vi "Write Motors with Encoders Config.vi"(8 "error in (no error)":errorcluster, 10 "Motors with Encoders Config":T1={"Counts  Per Revolution"=0, "Invert Encoder Direction"=FALSE, "Diameter of Revolution"=0.0, "Max RPM"=0.0, "Encoder Control"=TRUE}, 11 "Motors with Encoders in":refnum<class "Motors with Encoders.lvclass">) -> (0 "error out":errorcluster, 3 "Motors with Encoders out":refnum<class "Motors with Encoders.lvclass">)   [LabVIEW 2014, in "Motors with Encoders.lvlib" / "Motors with Encoders.lvclass"]
uses:
  Motors with Encoders.lvclass
  Motors with Encoders Config.ctl
  Motors with Encoders.lvclass/Motors with Encoders.ctl
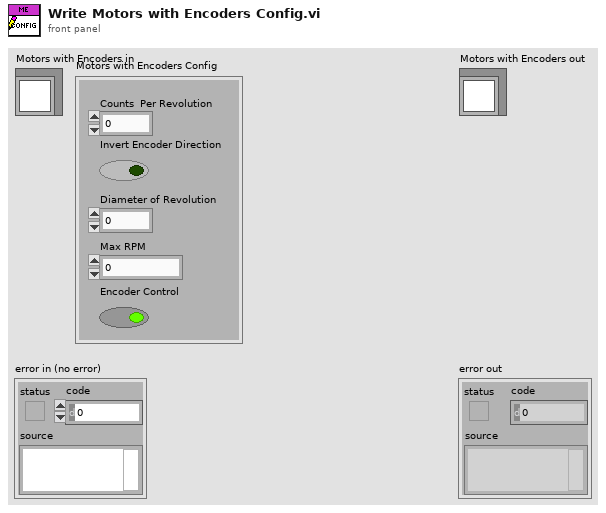
[diagram p1: front panel]
types:
  T1 = typedef "Motors with Encoders.lvlib/Motors with Encoders.lvclass/Motors with Encoders Config.ctl" = cluster{"Counts  Per Revolution":u32, "Invert Encoder Direction":bool, "Diameter of Revolution":dbl, "Max RPM":dbl, "Encoder Control":bool}
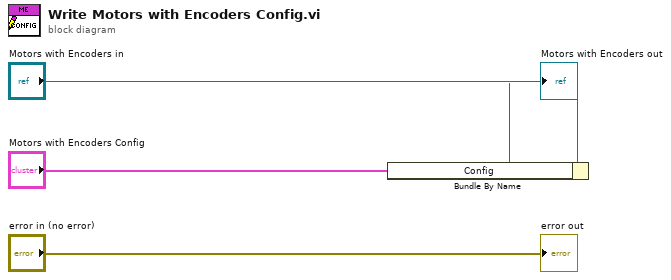
[diagram p0: block diagram]
diagram:
  n1 = Bundle By Name(cluster="Motors with Encoders in", "Config"="Motors with Encoders Config") -> (→"Motors with Encoders out":refnum<class "Motors with Encoders.lvclass">)
  "error out" <- "error in (no error)"
